vi "Receive_string.vi"(8 "error in":errorcluster, 9 "Flags":i16, 10 "buf in":string, 11 "socket in":refnum<class "Socket.lvclass">) -> (0 "error out":errorcluster, 2 "data":string, 3 "socket out":refnum<class "Socket.lvclass">)   [LabVIEW 2025, in "ZeroMQ.lvlib" / "Socket.lvclass"]
doc: "Receive a message from the socket and returns the received data as a LabVIEW string (which may contain NULL). If receiving a multi-part message, this VI must be called for each part of the message, and it is the user's obligation to check if this is required. Alternatively, use the zmq_recv_multi VI, which handles this automatically.\n\nIf <b>no block?</b> is True, the function call will return immediately. Use zmq_check_timeout to see if it was simply a timeout or an error occurred.\n\nOtherwise this call will block until a message is received, an error is raised, or the socket is closed.\n\nDetailed API documentation: http://api.zeromq.org/3-2:zmq-recv"
uses:
  Socket.lvclass
  Socket.lvclass/Socket.ctl
  libzmq-v143-mt-4_3_6/LibZMQ.lvlib
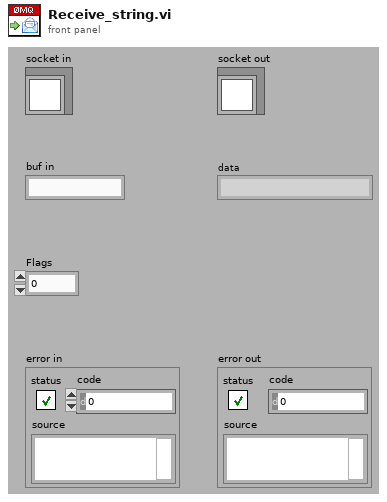
[diagram p1: front panel]
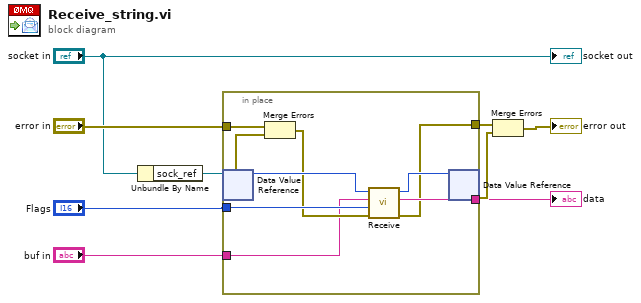
[diagram p0: block diagram]
diagram:
  n1 = Unbundle By Name("socket in") -> ("sock_ref"=w6:refnum<data-value>)
  n2 = in-place {
    in-place-border: "Flags" -> [w16]
    in-place-border: "error in" -> [w18]
    in-place-border: [w11] -> w8
    in-place-border: [w13] -> w3
    in-place-border: "buf in" -> [w10]
    n3 = in-place-dvr #1(w6) -> (w15:u64, w17:errorcluster)
    n4 = Merge Errors(w18, w17) -> (w12:errorcluster)
    n5 = call "Receive.vi"("error in (no error)"=w12, "flags_"=w16, "buf in"=w10, "s"=w15) -> ("error out"=w11:errorcluster, "buf out"=w13:string, "s_"=w14:u64)  [unwired: 5 in]
    n6 = in-place-dvr #1(w14) -> (w4:errorcluster)  [unwired: 1 out]
  }
  "data" <- w3
  n7 = Merge Errors(w8, w4) -> (→"error out":errorcluster)
  "socket out" <- "socket in"
